vi "Main Page.vi"(8 "error in (no error)":errorcluster, 11 "Node Ptr":T2 format="%.0x") -> (0 "error out":errorcluster)   [LabVIEW 2020, in "Waveform Analog Output System Explorer.lvlib"]
uses:
  Waveform Analog Output System Explorer.lvlib
  <vilib>/NI VeriStand/Custom Device API/Custom Device Item Ref.ctl
  Number of AO Channels.ctl
  Shared/Constants.vi
  <vilib>/NI VeriStand/Custom Device API/Get Item Property (Double).vi
  <vilib>/NI VeriStand/Custom Device API/Set Item Property (Double).vi
  <vilib>/NI VeriStand/Custom Device API/Get Item Property (U32).vi
  <vilib>/NI VeriStand/Custom Device API/Set Item Property (U32).vi
  <vilib>/NI VeriStand/Custom Device API/Get Item Property (I32).vi
  <vilib>/NI VeriStand/Custom Device API/Set Item Property (I32).vi
  <vilib>/NI VeriStand/Custom Device API/Get Item Property (String).vi
  <vilib>/NI VeriStand/Custom Device API/Get Item Property (U16).vi
  <vilib>/NI VeriStand/Custom Device API/Get Item Property (Variant).vi
  <vilib>/NI VeriStand/Custom Device API/Set Item Property (String).vi
  <vilib>/NI VeriStand/Custom Device API/Set Item Property (U16).vi
  <vilib>/NI VeriStand/Custom Device API/Set Item Property (Variant).vi
  <vilib>/NI VeriStand/Custom Device API/Custom Device API.lvlib
  Shared/Waveform Analog Output Shared.lvlib
panel:
  in  "# L2 Buffers":i32=-1
  out "WF Parameters Update Rate (Hz)":dbl caption="WF Parameters Update Rate (Hz)\nUpdate Rate (Hz) = Sample Rate (Hz) / # Samples"
  in  "Data Loop Update Interval (ms)":u32=100 caption="*****  MUST MATCH *****\nData Loop Update Interval (ms)\nInterval (ms) = 1000 * # Samples / Sample Rate (Hz)"
  in  "# AO Channels":T1=8 items=["2 chs"=2, "4 chs"=4, "8 chs"=8, "32 chs"=32, "64 chs"=64]
  in  "# L1 Buffers":i32=2
  in  "Start Delay (s)":dbl
  in  "# Samples":dbl=1000.0
  in  "Sample Rate (Hz)":dbl=10000.0
  in  "Min Voltage (V)":dbl=-10.0
  in  "Max Voltage (V)":dbl=10.0
  in  "DAQ Name":string caption="DAQ Device Name (Ex: PXI1Slot2)"
  in  "Configure Physical Channels":bool
  in  "Header":cluster{"Section Name":string}={"Section Name"="Waveform Analog Output Configuration"}
  in  "Description":string
  in  "Name":string
  # "Device Settings"
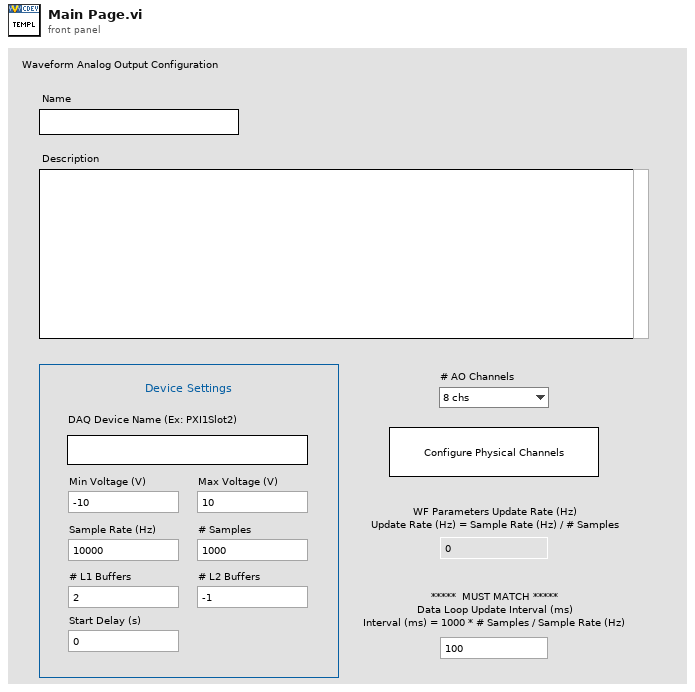
[diagram p1: front panel]
types:
  T1 = typedef "Waveform Analog Output System Explorer.lvlib/Number of AO Channels.ctl" = u16
  T2 = typedef "Custom Device API.lvlib/Custom Device Item Ref.ctl" = u64
  T3 = typedef "Custom Device API.lvlib/Custom Device Item Info.ctl" = cluster{"Name":string, "Is Channel":bool, "GUID":string, "Is Waveform":bool}
  T4 = typedef "Custom Device API.lvlib/Custom Device Commands.ctl" = enum16{"Default", "Item renamed", "Shutdown", "Dynamic button pressed"}
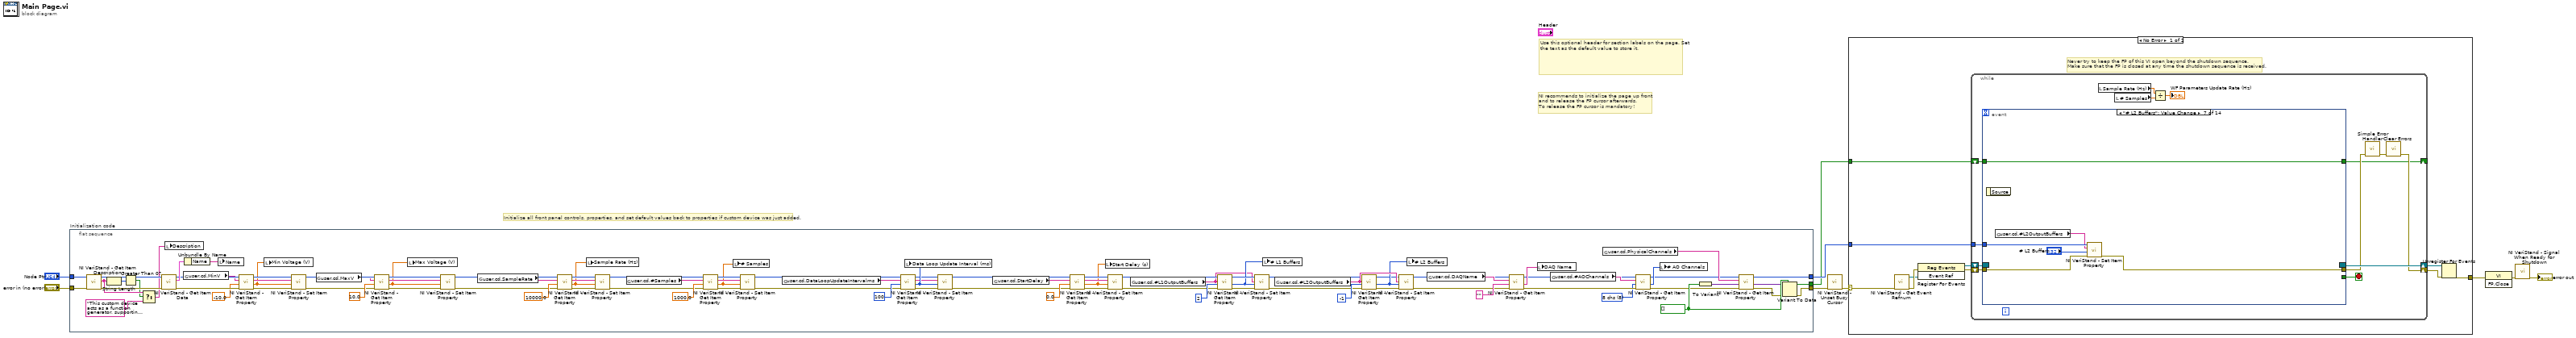
[diagram p0: block diagram]
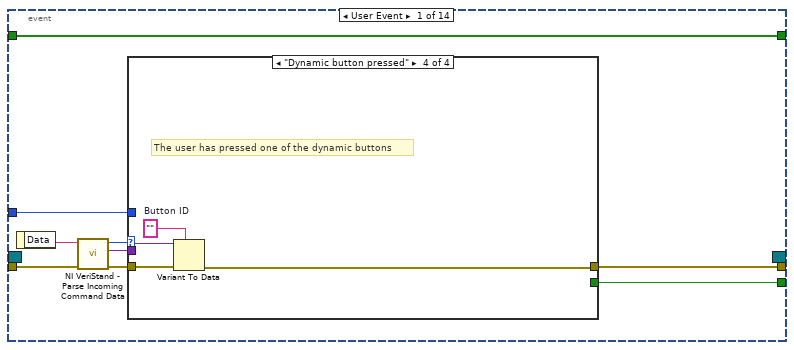
[diagram p2: hidden frame]
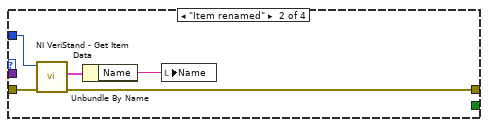
[diagram p4: hidden frame]
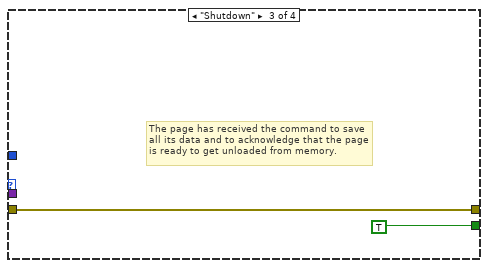
[diagram p5: hidden frame]
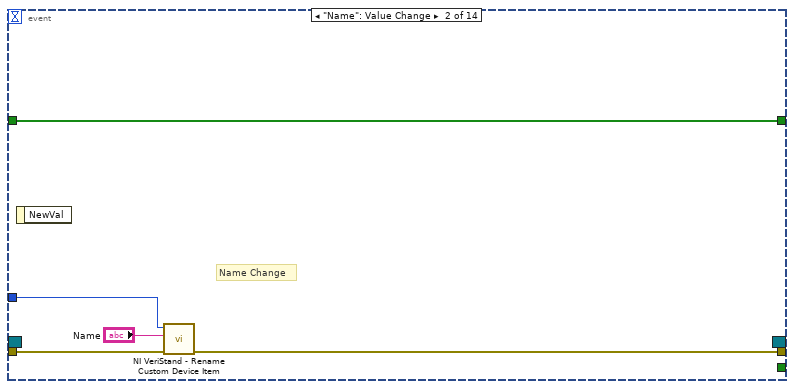
[diagram p6: hidden frame]
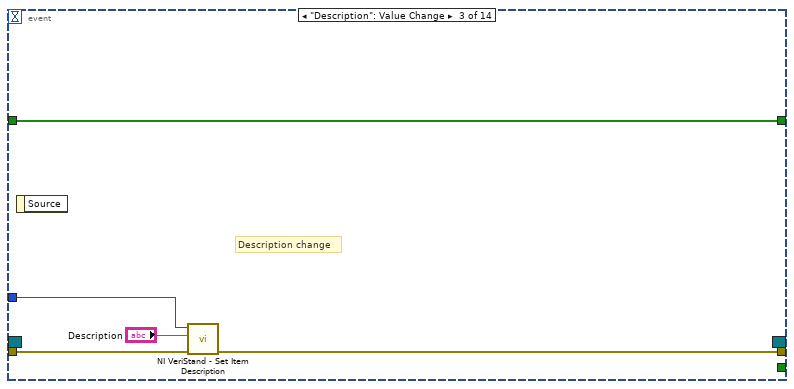
[diagram p7: hidden frame]
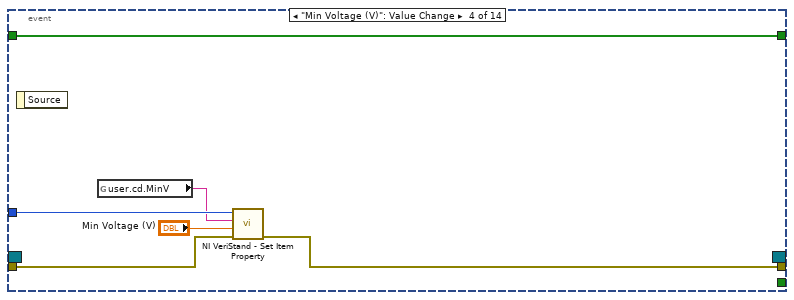
[diagram p8: hidden frame]
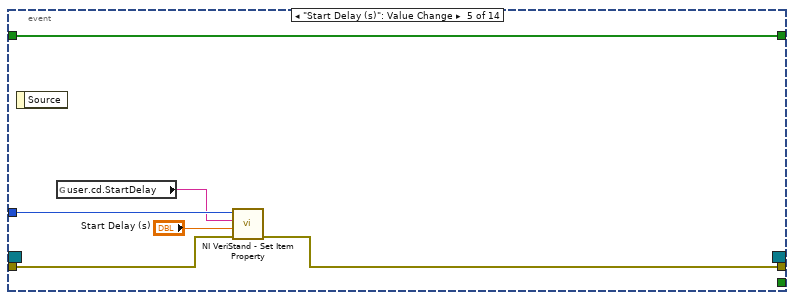
[diagram p9: hidden frame]
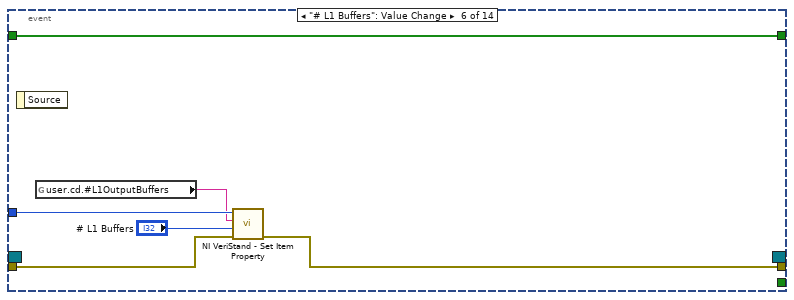
[diagram p10: hidden frame]
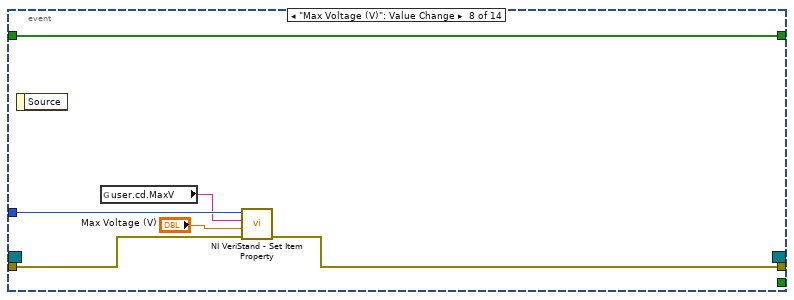
[diagram p11: hidden frame]
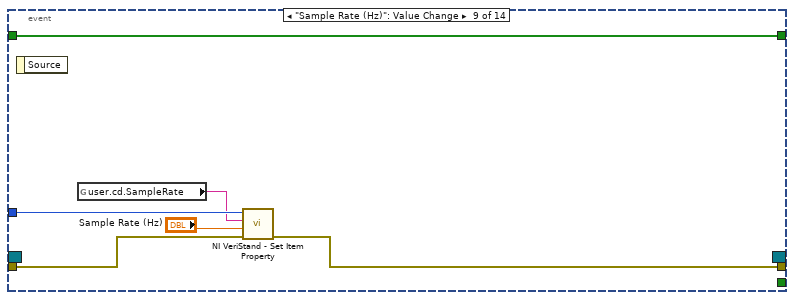
[diagram p12: hidden frame]
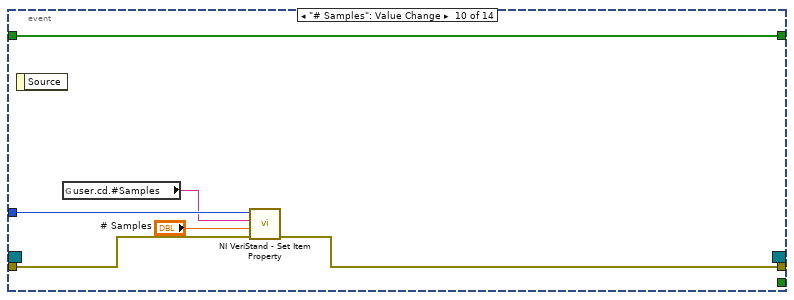
[diagram p13: hidden frame]
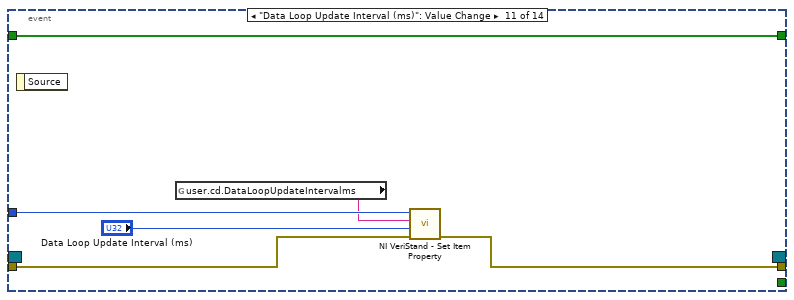
[diagram p14: hidden frame]
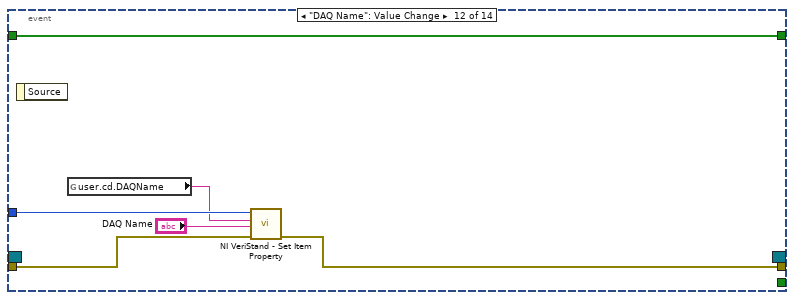
[diagram p15: hidden frame]
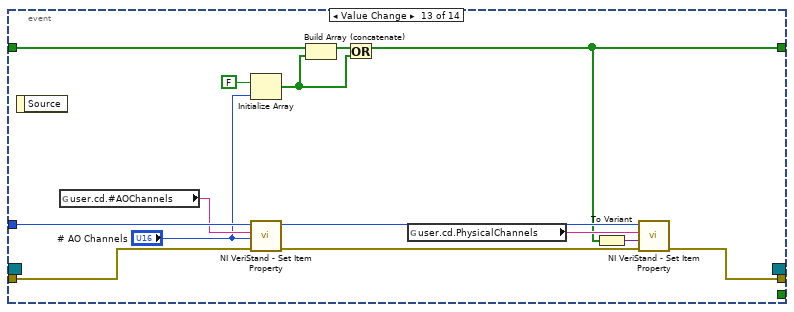
[diagram p16: hidden frame]
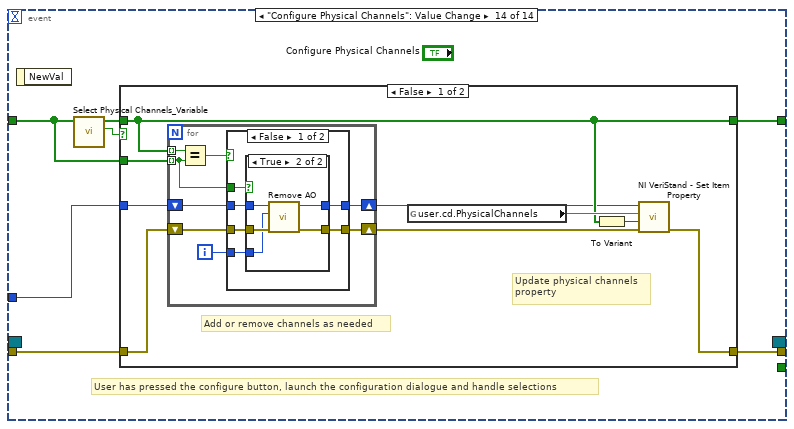
[diagram p17: hidden frame]
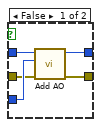
[diagram p18: hidden frame]
diagram:
  # "Initialize all front panel controls, properties, and set default values back to properties if custom device was just added."
  # "Use this optional header for section labels on the page. Set the text as the default value to store it."
  # "NI recommends to initialize the page up front\nand to release the FP cursor afterwards.\nTo release the FP cursor is mandatory!"
  n1 = flat-sequence "Initialization code" {
    tunnel: "error in (no error)" -> [w95]
    tunnel: "Node Ptr" -> [w94]
    tunnel: [w36] -> w5
    tunnel: [w37] -> w2
    tunnel: [w38] -> w1
    frame #0 {
      w29 = T1 8 items=["2 chs"=2, "4 chs"=4, "8 chs"=8, "32 chs"=32, "64 chs"=64] ("Number of AO Channels 2")
      w79 = bool[] []
      n2 = call <vilib>:"NI VeriStand - Get Item Description.vi"("error in (no error)"=w95, "Item Ref in"=w94) -> ("error out"=w93:errorcluster, "Description"=w53:string, "Item Ref out"=w96:T2)  [unwired: 7 out]
      n3 = String Length(string=w53) -> (length=w54:i32)
      n4 = Greater Than 0?(x=w54) -> (x > 0?=w52:bool)
      n5 = Select(t=w53, s=w52, f="This custom device acts as a function generator, supporting the generation of sine, square, triangle, and sawtooth waveforms. To use this custom device, complete the following:\n1. Enter configuration data below for DAQ name, voltage range, and sampling info.\n2. Press the \"Configure Physical Channels\" button to add or remove AO channels.\n3. Expand the AO# sections to see the tuning channels that are available.  " ("Description")) -> (s? t:f=w55:string)
      n6 = call <vilib>:"NI VeriStand - Get Item Data.vi"("error in (no error)"=w93, "Item Ref in"=w96) -> ("error out"=w89:errorcluster, "Item Info"=w92:T3, "Item Ref out"=w90:T2)  [unwired: 7 out]
      n7 = local write "Description"(w55) -> ()
      n8 = global read "Constants.vi" "user.cd.MinV"() -> (w75:string)
      n9 = Unbundle By Name(w92) -> ("Name"=w91:string)
      n10 = local write "Name"(w91) -> ()
      n11 = call-poly <vilib>:"NI VeriStand - Get Item Property.vi"("error in (no error)"=w89, "Default Value"=-10.0, "Property Name"=w75, "Item Ref in"=w90) -> ("error out"=w73:errorcluster, "Value"=w74:dbl, "Item Ref out"=w76:T2)  [unwired: 4 in, 1 out]
      n12 = local write "Min Voltage (V)"(w74) -> ()
      n13 = call-poly <vilib>:"NI VeriStand - Set Item Property.vi"("error in (no error)"=w73, "Value"=w74, "Property Name"=w75, "Item Ref in"=w76) -> ("error out"=w72:errorcluster, "Item Ref out"=w71:T2)  [unwired: 5 in, 1 out]
      n14 = global read "Constants.vi" "user.cd.MaxV"() -> (w67:string)
      n15 = call-poly <vilib>:"NI VeriStand - Get Item Property.vi"("error in (no error)"=w72, "Default Value"=10.0, "Property Name"=w67, "Item Ref in"=w71) -> ("error out"=w85:errorcluster, "Value"=w66:dbl, "Item Ref out"=w69:T2)  [unwired: 4 in, 1 out]
      n16 = local write "Max Voltage (V)"(w66) -> ()
      n17 = call-poly <vilib>:"NI VeriStand - Set Item Property.vi"("error in (no error)"=w85, "Value"=w66, "Property Name"=w67, "Item Ref in"=w69) -> ("error out"=w70:errorcluster, "Item Ref out"=w68:T2)  [unwired: 5 in, 1 out]
      n18 = global read "Constants.vi" "user.cd.SampleRate"() -> (w64:string)
      n19 = call-poly <vilib>:"NI VeriStand - Get Item Property.vi"("error in (no error)"=w70, "Default Value"=10000.0, "Property Name"=w64, "Item Ref in"=w68) -> ("error out"=w84:errorcluster, "Value"=w63:dbl, "Item Ref out"=w65:T2)  [unwired: 4 in, 1 out]
      n20 = local write "Sample Rate (Hz)"(w63) -> ()
      n21 = call-poly <vilib>:"NI VeriStand - Set Item Property.vi"("error in (no error)"=w84, "Value"=w63, "Property Name"=w64, "Item Ref in"=w65) -> ("error out"=w58:errorcluster, "Item Ref out"=w59:T2)  [unwired: 5 in, 1 out]
      n22 = global read "Constants.vi" "user.cd.#Samples"() -> (w57:string)
      n23 = call-poly <vilib>:"NI VeriStand - Get Item Property.vi"("error in (no error)"=w58, "Default Value"=1000.0, "Property Name"=w57, "Item Ref in"=w59) -> ("error out"=w61:errorcluster, "Value"=w56:dbl, "Item Ref out"=w62:T2)  [unwired: 4 in, 1 out]
      n24 = local write "# Samples"(w56) -> ()
      n25 = call-poly <vilib>:"NI VeriStand - Set Item Property.vi"("error in (no error)"=w61, "Value"=w56, "Property Name"=w57, "Item Ref in"=w62) -> ("error out"=w21:errorcluster, "Item Ref out"=w23:T2)  [unwired: 5 in, 1 out]
      n26 = global read "Constants.vi" "user.cd.DataLoopUpdateIntervalms"() -> (w27:string)
      n27 = call-poly <vilib>:"NI VeriStand - Get Item Property.vi"("error in (no error)"=w21, "Default Value"=u32 100, "Property Name"=w27, "Item Ref in"=w23) -> ("error out"=w25:errorcluster, "Value"=w28:u32, "Item Ref out"=w24:T2)  [unwired: 4 in, 1 out]
      n28 = local write "Data Loop Update Interval (ms)"(w28) -> ()
      n29 = call-poly <vilib>:"NI VeriStand - Set Item Property.vi"("error in (no error)"=w25, "Value"=w28, "Property Name"=w27, "Item Ref in"=w24) -> ("error out"=w20:errorcluster, "Item Ref out"=w22:T2)  [unwired: 5 in, 1 out]
      n30 = global read "Constants.vi" "user.cd.StartDelay"() -> (w50:string)
      n31 = call-poly <vilib>:"NI VeriStand - Get Item Property.vi"("error in (no error)"=w20, "Default Value"=0.0, "Property Name"=w50, "Item Ref in"=w22) -> ("error out"=w48:errorcluster, "Value"=w46:dbl, "Item Ref out"=w47:T2)  [unwired: 4 in, 1 out]
      n32 = local write "Start Delay (s)"(w46) -> ()
      n33 = call-poly <vilib>:"NI VeriStand - Set Item Property.vi"("error in (no error)"=w48, "Value"=w46, "Property Name"=w50, "Item Ref in"=w47) -> ("error out"=w41:errorcluster, "Item Ref out"=w42:T2)  [unwired: 5 in, 1 out]
      n34 = global read "Constants.vi" "user.cd.#L1OutputBuffers"() -> (w19:string)
      n35 = call-poly <vilib>:"NI VeriStand - Get Item Property.vi"("error in (no error)"=w41, "Default Value"=2, "Property Name"=w19, "Item Ref in"=w42) -> ("error out"=w44:errorcluster, "Value"=w40:i32, "Item Ref out"=w45:T2)  [unwired: 4 in, 1 out]
      n36 = call-poly <vilib>:"NI VeriStand - Set Item Property.vi"("error in (no error)"=w44, "Value"=w40, "Property Name"=w19, "Item Ref in"=w45) -> ("error out"=w13:errorcluster, "Item Ref out"=w11:T2)  [unwired: 5 in, 1 out]
      n37 = local write "# L1 Buffers"(w40) -> ()
      n38 = global read "Constants.vi" "user.cd.#L2OutputBuffers"() -> (w18:string)
      n39 = call-poly <vilib>:"NI VeriStand - Get Item Property.vi"("error in (no error)"=w13, "Default Value"=-1, "Property Name"=w18, "Item Ref in"=w11) -> ("error out"=w15:errorcluster, "Value"=w17:i32, "Item Ref out"=w14:T2)  [unwired: 4 in, 1 out]
      n40 = call-poly <vilib>:"NI VeriStand - Set Item Property.vi"("error in (no error)"=w15, "Value"=w17, "Property Name"=w18, "Item Ref in"=w14) -> ("error out"=w12:errorcluster, "Item Ref out"=w10:T2)  [unwired: 5 in, 1 out]
      n41 = local write "# L2 Buffers"(w17) -> ()
      n42 = global read "Constants.vi" "user.cd.DAQName"() -> (w82:string)
      n43 = call-poly <vilib>:"NI VeriStand - Get Item Property.vi"("error in (no error)"=w12, "Default Value"="", "Property Name"=w82, "Item Ref in"=w10) -> ("error out"=w31:errorcluster, "Value"=w80:string, "Item Ref out"=w33:T2)  [unwired: 4 in, 1 out]
      n44 = local write "DAQ Name"(w80) -> ()
      n45 = global read "Constants.vi" "user.cd.#AOChannels"() -> (w34:string)
      n46 = global read "Constants.vi" "user.cd.PhysicalChannels"() -> (w39:string)
      n47 = call-poly <vilib>:"NI VeriStand - Get Item Property.vi"("error in (no error)"=w31, "Default Value"=w29, "Property Name"=w34, "Item Ref in"=w33) -> ("error out"=w30:errorcluster, "Value"=w35:u16, "Item Ref out"=w32:T2)  [unwired: 4 in, 1 out]
      n48 = local write "# AO Channels"(w35) -> ()
      n49 = To Variant(anything=w79) -> (Variant=w83:variant)
      n50 = call-poly <vilib>:"NI VeriStand - Get Item Property.vi"("error in (no error)"=w30, "Default Value"=w83, "Property Name"=w39, "Item Ref in"=w32) -> ("error out"=w78:errorcluster, "Value"=w77:variant, "Item Ref out"=w37:T2)  [unwired: 4 in, 1 out]
      n51 = Variant To Data(error in=w78, type=w79, Variant=w77) -> (data=w38:bool[], error out=w36:errorcluster)
    }
  }
  n52 = call <vilib>:"NI VeriStand - Unset Busy Cursor.vi"("error in (no error)"=w5) -> ("error out"=w4:errorcluster)  [unwired: 10 out]
  n53 = case shown="No Error" w4 {
    selector: w4 -> [w98 w265]
    tunnel: [w103 w263] -> w9
    tunnel: w2 -> [w99 _]
    tunnel: w1 -> [w97 _]
    frame No Error {
      # "Never try to keep the FP of this VI open beyond the shutdown sequence.\nMake sure that the FP is closed at any time the shutdown sequence is received."
      n54 = call <vilib>:"NI VeriStand - Get Event Refnum.vi"("error in (no error)"=w98) -> ("error out"=w106:errorcluster, "Event Ref"=w102:refnum<user-event>)  [unwired: 9 out]
      n55 = register-events(error in=w106, w102) -> (reference out=w100:refnum<event-registration>, error out=w101:errorcluster)  [unwired: 1 in]
      n56 = while {
        tunnel: w99 -> [w115]
        shift-right: [w112] -> w104
        shift-left: w101 -> [w118]
        shift-right: [w119] -> w105
        shift-left: w100 -> [w117]
        shift-right: [w110] -> _
        shift-left: w97 -> [w111]
        stop <- w116 stop-if-true
        n57 = event shown="[6] \"# L2 Buffers\": Value Change" {
          selector: w117 -> [_ _ _ _ _ _ _ _ _ _ _ _ _ _]
          dyn-events: [_ _ _ _ _ _ _ _ _ _ _ _ _ _] -> w119
          timeout: _ -> [_ _ _ _ _ _ _ _ _ _ _ _ _ _]
          tunnel: w118 -> [w128 w145 w149 w155 w161 w167 w173 w179 w185 w191 w197 w203 w217 w225]
          tunnel: [w124 _ _ _ _ _ _ _ _ _ _ _ _ _] -> w116
          tunnel: [w123 w144 w148 w152 w159 w166 w172 w177 w183 w189 w195 w201 w209 w224] -> w114
          tunnel: w115 -> [w122 w143 w150 w156 w162 w168 w174 w180 w186 w192 w198 w204 w218 w223]
          tunnel: w111 -> [w120 w141 w146 w151 w158 w165 w171 w175 w181 w188 w194 w200 w215 w219]
          tunnel: [w120 w141 w146 w151 w158 w165 w171 w175 w181 w188 w194 w200 w206 w221] -> w110
          event User Event {
            n58 = event-data() -> ("Data"=w127:string)  [unwired: 1 out]
            n59 = call <vilib>:"NI VeriStand - Parse Incoming Command Data.vi"("error in (no error)"=w128, "Incoming data"=w127) -> ("error out"=w126:errorcluster, "Outgoing data"=w121:variant, "Action"=w125:T4)  [unwired: 7 out]
            n60 = case shown="\"Dynamic button pressed\"" w125 {
              tunnel: w126 -> [w129 w134 w135 w140]
              tunnel: [_ _ TRUE _] -> w124
              tunnel: [w129 w131 w135 w137] -> w123
              tunnel: w122 -> [_ w133 _ _]
              tunnel: w121 -> [_ _ _ w139]
              frame "Default", Default {
              }
              frame "Item renamed" {
                n61 = call <vilib>:"NI VeriStand - Get Item Data.vi"("error in (no error)"=w134, "Item Ref in"=w133) -> ("error out"=w131:errorcluster, "Item Info"=w132:T3)  [unwired: 8 out]
                n62 = Unbundle By Name(w132) -> ("Name"=w130:string)
                n63 = local write "Name"(w130) -> ()
              }
              frame "Shutdown" {
                # "The page has received the command to save all its data and to acknowledge that the page is ready to get unloaded from memory."
              }
              frame "Dynamic button pressed" {
                w138 = ""  # Button ID
                # "The user has pressed one of the dynamic buttons"
                n64 = Variant To Data(error in=w140, type=w138, Variant=w139) -> (error out=w137:errorcluster)  [unwired: 1 out]
              }
            }
          }
          event "Name": Value Change {
            # "Name Change"
            n65 = event-data() -> ()  [unwired: 2 out]
            n66 = call <vilib>:"NI VeriStand - Rename Custom Device Item.vi"("error in (no error)"=w145, "New Name"="Name", "Item Ref in"=w143) -> ("error out"=w144:errorcluster)  [unwired: 1 in, 7 out]
          }
          event "Description": Value Change {
            # "Description change"
            n67 = event-data() -> ()  [unwired: 2 out]
            n68 = call <vilib>:"NI VeriStand - Set Item Description.vi"("error in (no error)"=w149, "Description"="Description", "Item Ref in"=w150) -> ("error out"=w148:errorcluster)  [unwired: 8 out]
          }
          event "Min Voltage (V)": Value Change {
            n69 = event-data() -> ()  [unwired: 2 out]
            n70 = global read "Constants.vi" "user.cd.MinV"() -> (w154:string)
            n71 = call-poly <vilib>:"NI VeriStand - Set Item Property.vi"("error in (no error)"=w155, "Value"="Min Voltage (V)", "Property Name"=w154, "Item Ref in"=w156) -> ("error out"=w152:errorcluster)  [unwired: 5 in, 2 out]
          }
          event "Start Delay (s)": Value Change {
            n72 = event-data() -> ()  [unwired: 2 out]
            n73 = global read "Constants.vi" "user.cd.StartDelay"() -> (w160:string)
            n74 = call-poly <vilib>:"NI VeriStand - Set Item Property.vi"("error in (no error)"=w161, "Value"="Start Delay (s)", "Property Name"=w160, "Item Ref in"=w162) -> ("error out"=w159:errorcluster)  [unwired: 5 in, 2 out]
          }
          event "# L1 Buffers": Value Change {
            n75 = event-data() -> ()  [unwired: 2 out]
            n76 = global read "Constants.vi" "user.cd.#L1OutputBuffers"() -> (w163:string)
            n77 = call-poly <vilib>:"NI VeriStand - Set Item Property.vi"("error in (no error)"=w167, "Value"="# L1 Buffers", "Property Name"=w163, "Item Ref in"=w168) -> ("error out"=w166:errorcluster)  [unwired: 5 in, 2 out]
          }
          event "# L2 Buffers": Value Change {
            n78 = event-data() -> ()  [unwired: 2 out]
            n79 = global read "Constants.vi" "user.cd.#L2OutputBuffers"() -> (w170:string)
            n80 = call-poly <vilib>:"NI VeriStand - Set Item Property.vi"("error in (no error)"=w173, "Value"="# L2 Buffers", "Property Name"=w170, "Item Ref in"=w174) -> ("error out"=w172:errorcluster)  [unwired: 5 in, 2 out]
          }
          event "Max Voltage (V)": Value Change {
            n81 = event-data() -> ()  [unwired: 2 out]
            n82 = global read "Constants.vi" "user.cd.MaxV"() -> (w178:string)
            n83 = call-poly <vilib>:"NI VeriStand - Set Item Property.vi"("error in (no error)"=w179, "Value"="Max Voltage (V)", "Property Name"=w178, "Item Ref in"=w180) -> ("error out"=w177:errorcluster)  [unwired: 5 in, 2 out]
          }
          event "Sample Rate (Hz)": Value Change {
            n84 = event-data() -> ()  [unwired: 2 out]
            n85 = global read "Constants.vi" "user.cd.SampleRate"() -> (w184:string)
            n86 = call-poly <vilib>:"NI VeriStand - Set Item Property.vi"("error in (no error)"=w185, "Value"="Sample Rate (Hz)", "Property Name"=w184, "Item Ref in"=w186) -> ("error out"=w183:errorcluster)  [unwired: 5 in, 2 out]
          }
          event "# Samples": Value Change {
            n87 = event-data() -> ()  [unwired: 2 out]
            n88 = global read "Constants.vi" "user.cd.#Samples"() -> (w190:string)
            n89 = call-poly <vilib>:"NI VeriStand - Set Item Property.vi"("error in (no error)"=w191, "Value"="# Samples", "Property Name"=w190, "Item Ref in"=w192) -> ("error out"=w189:errorcluster)  [unwired: 5 in, 2 out]
          }
          event "Data Loop Update Interval (ms)": Value Change {
            n90 = event-data() -> ()  [unwired: 2 out]
            n91 = global read "Constants.vi" "user.cd.DataLoopUpdateIntervalms"() -> (w196:string)
            n92 = call-poly <vilib>:"NI VeriStand - Set Item Property.vi"("error in (no error)"=w197, "Value"="Data Loop Update Interval (ms)", "Property Name"=w196, "Item Ref in"=w198) -> ("error out"=w195:errorcluster)  [unwired: 5 in, 2 out]
          }
          event "DAQ Name": Value Change {
            n93 = event-data() -> ()  [unwired: 2 out]
            n94 = global read "Constants.vi" "user.cd.DAQName"() -> (w202:string)
            n95 = call-poly <vilib>:"NI VeriStand - Set Item Property.vi"("error in (no error)"=w203, "Value"="DAQ Name", "Property Name"=w202, "Item Ref in"=w204) -> ("error out"=w201:errorcluster)  [unwired: 5 in, 2 out]
          }
          event Value Change {
            n96 = event-data() -> ()  [unwired: 2 out]
            n97 = global read "Constants.vi" "user.cd.#AOChannels"() -> (w216:string)
            n98 = Initialize Array(FALSE, "# AO Channels") -> (w205:bool[])
            n99 = call-poly <vilib>:"NI VeriStand - Set Item Property.vi"("error in (no error)"=w217, "Value"="# AO Channels", "Property Name"=w216, "Item Ref in"=w218) -> ("error out"=w211:errorcluster, "Item Ref out"=w212:T2)  [unwired: 5 in, 1 out]
            n100 = Build Array (concatenate)(w215, w205) -> (w210:bool[])
            n101 = Or(x=w210, y=w205) -> (x .or. y?=w206:bool[])
            n102 = global read "Constants.vi" "user.cd.PhysicalChannels"() -> (w214:string)
            n103 = To Variant(anything=w206) -> (Variant=w213:variant)
            n104 = call-poly <vilib>:"NI VeriStand - Set Item Property.vi"("error in (no error)"=w211, "Value"=w213, "Property Name"=w214, "Item Ref in"=w212) -> ("error out"=w209:errorcluster)  [unwired: 5 in, 2 out]
          }
          event "Configure Physical Channels": Value Change {
            # "User has pressed the configure button, launch the configuration dialogue and handle selections"
            n105 = event-data() -> ()  [unwired: 2 out]
            n106 = call "Select Physical Channels_Variable.vi"("Physical Channels In"=w219) -> ("Cancelled?"=w220:bool, "Physical Channels Out"=w222:bool[])  [unwired: 8 in, 1 out]
            n107 = case shown="False" w220 {
              tunnel: w225 -> [w227 w261]
              tunnel: [w234 w261] -> w224
              tunnel: w223 -> [w229 _]
              tunnel: w222 -> [w231 w262]
              tunnel: [w231 w262] -> w221
              tunnel: w219 -> [w230 _]
              frame False {
                # "Update physical channels\nproperty"
                # "Add or remove channels as needed"
                n108 = for {
                  tunnel: w231 -> [w242] mode=indexing
                  tunnel: w230 -> [w238] mode=indexing
                  shift-right: [w236] -> w228
                  shift-left: w229 -> [w240]
                  shift-right: [w235] -> w226
                  shift-left: w227 -> [w239]
                  i -> [w237]
                  n109 = Equal?(x=w242, y=w238) -> (x = y?=w241:bool)
                  n110 = case shown="False" w241 {
                    tunnel: w240 -> [w246 w260]
                    tunnel: w239 -> [w245 w259]
                    tunnel: w238 -> [w248 _]
                    tunnel: w237 -> [w247 _]
                    tunnel: [w244 w260] -> w236
                    tunnel: [w243 w259] -> w235
                    frame False {
                      n111 = case shown="True" w248 {
                        tunnel: w247 -> [w252 w257]
                        tunnel: w246 -> [w253 w256]
                        tunnel: w245 -> [w251 w258]
                        tunnel: [w250 w254] -> w244
                        tunnel: [w249 w255] -> w243
                        frame False {
                          n112 = call "Add AO.vi"("error in (no error)"=w251, "Physical Channel Number"=w252, "Device Item Ref in"=w253) -> ("error out"=w249:errorcluster, "Parent Ref out"=w250:T2)  [unwired: 7 in]
                        }
                        frame True {
                          n113 = call "Remove AO.vi"("error in (no error)"=w258, "Iteration"=w257, "Item Ref in"=w256) -> ("error out"=w255:errorcluster, "Item Ref out"=w254:T2)  [unwired: 7 in]
                        }
                      }
                    }
                    frame True {
                    }
                  }
                }
                n114 = global read "Constants.vi" "user.cd.PhysicalChannels"() -> (w233:string)
                n115 = To Variant(anything=w231) -> (Variant=w232:variant)
                n116 = call-poly <vilib>:"NI VeriStand - Set Item Property.vi"("error in (no error)"=w226, "Value"=w232, "Property Name"=w233, "Item Ref in"=w228) -> ("error out"=w234:errorcluster)  [unwired: 5 in, 2 out]
              }
              frame True {
              }
            }
          }
        }
        n117 = local read "Sample Rate (Hz)"() -> (w109:dbl)
        n118 = local read "# Samples"() -> (w108:dbl)
        n119 = Divide(x=w109, y=w108) -> (x/y=→"WF Parameters Update Rate (Hz)":dbl)
        n120 = call <vilib>:"Simple Error Handler.vi"("error in (no error)"=w114) -> ("error out"=w113:errorcluster)  [unwired: 1 in, 7 out]
        n121 = call <vilib>:"Clear Errors.vi"("error in (no error)"=w113) -> ("error out"=w112:errorcluster)  [unwired: 1 in, 5 out]
      }
      n122 = Unregister For Events(event registration refnum=w105, error in=w104) -> (error out=w103:errorcluster)
    }
    frame Error {
      n123 = call <vilib>:"Simple Error Handler.vi"("error in (no error)"=w265) -> ("error out"=w264:errorcluster)  [unwired: 1 in, 7 out]
      n124 = call <vilib>:"Clear Errors.vi"("error in (no error)"=w264) -> ("error out"=w263:errorcluster)  [unwired: 1 in, 5 out]
    }
  }
  n125 = invoke class="VI" method="FP.Close"(error in=w9) -> (error out=w8:errorcluster)  [unwired: 2 in, 2 out]
  n126 = call <vilib>:"NI VeriStand - Signal When Ready for Shutdown.vi"("error in (no error)"=w8) -> ("error out"=→"error out":errorcluster)  [unwired: 10 out]
